vi "Script Find current Constants.vi"(8 "error in":errorcluster, 11 "Library in":refnum<vi>) -> (0 "error out":errorcluster, 1 "All Constant VIS":path[](array[path]), 2 "Constants Info":T1[](array[typedef]), 3 "Library out":refnum<vi>)   [LabVIEW 2020, in "ConstantErrorsMaker.lvlib"]
uses:
  ConstantErrorsMaker.lvlib
  Constant Info--cluster.ctl
  <vilib>/Utility/traverseref.llb/TRef TravTarget.ctl
  <vilib>/Utility/traverseref.llb/VI Scripting - Traverse.lvlib
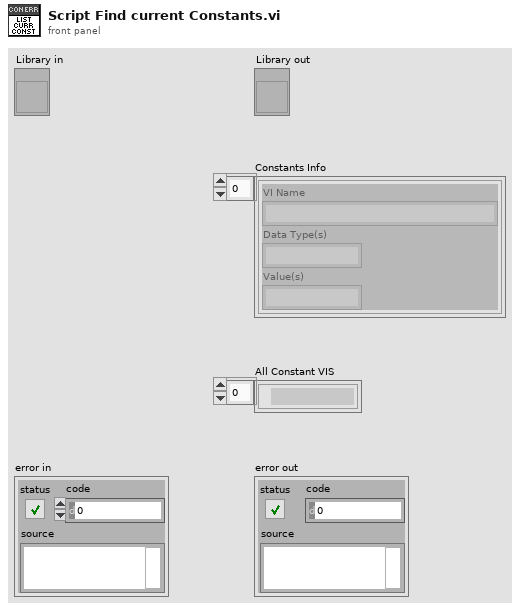
[diagram p1: front panel]
types:
  T1 = typedef "ConstantErrorsMaker.lvlib/Constant Info--cluster.ctl" = cluster{"VI Name":string, "Data Type(s)":string, "Value(s)":string}
  T2 = typedef "TRef TravTarget.ctl" = enum16{"FP", "BD", "Other"}
  T3 = typedef "NI_Data Type.lvlib/Data Type.ctl" = enum8{"Invalid Type", "Void", "I8", "I16", "I32", "I64", "U8", "U16", "U32", "U64", "Single Float", "Double Float", "Extended Float", "Single Complex", "Double Complex", "Extended Complex", "Enum U8", "Enum U16", "Enum U32", "Enum U64", "Single Float With Unit", "Double Float With Unit", "Extended Float With Unit", "Single Complex with Unit", "Double Complex with Unit", "Extended Complex with Unit", "Boolean", "String", "Path", "Picture", "Tag", "Array", "Cluster", "Variant", "LV Variant", "Waveform", "Timestamp", "Digital Waveform", "Digital Data", "ExpressData", "Refnum", "External Data", "VI", "Poly VI", "LabVIEW Class Instance", "Fixed Point", "Set Collection", "Map Collection"}
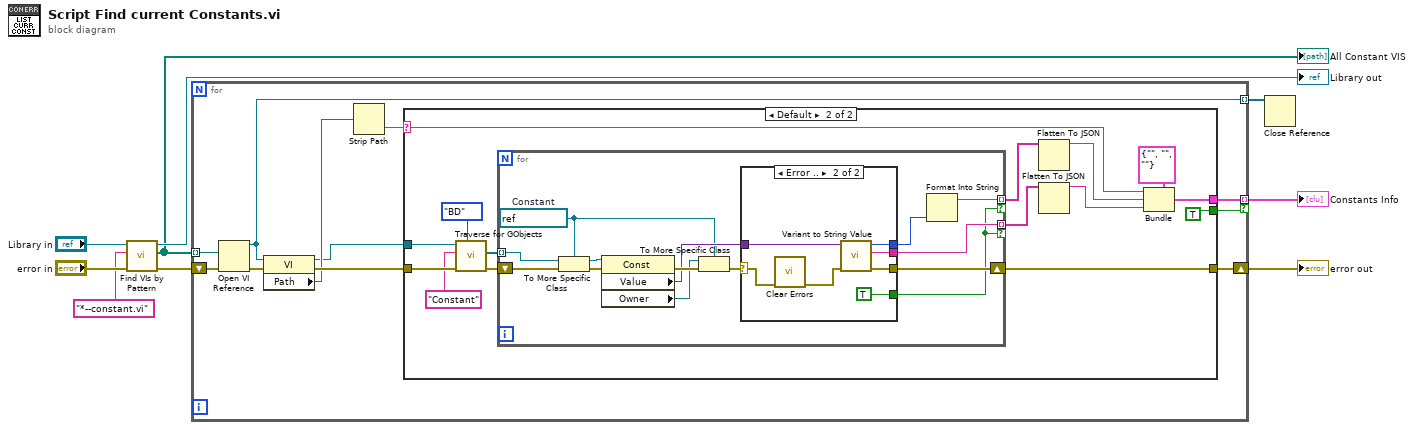
[diagram p0: block diagram]
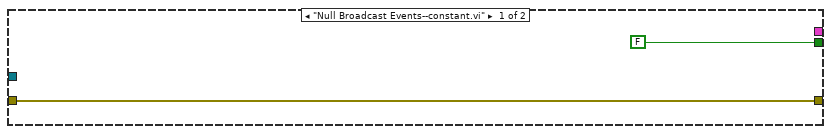
[diagram p2: hidden frame]
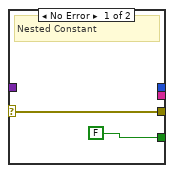
[diagram p3: hidden frame]
diagram:
  n1 = call "Find VIs by Pattern.vi"("error in"="error in", "pattern"="*--constant.vi", "Library in"="Library in") -> ("error out"=w7:errorcluster, "All Files in Dir"=w3:path[], "Library out"=→"Library out":refnum<vi>)  [unwired: 6 in]
  "All Constant VIS" <- w3
  n2 = for {
    tunnel: w3 -> [w16] mode=indexing
    shift-right: [w18] -> w8
    shift-left: w7 -> [w17]
    tunnel: [w12] -> w1 mode=indexing if=w10
    tunnel: [w11] -> w2 mode=indexing
    n3 = Open VI Reference(vi path=w16, error in (no error)=w17) -> (vi reference=w11:refnum<vi>, error out=w19:errorcluster)  [unwired: 4 in]
    n4 = property class="VI"(reference=w11, error in=w19) -> (reference out=w13:refnum<vi>, error out=w20:errorcluster, "Path"=w14:path)
    n5 = Strip Path(path=w14) -> (name=w15:string)  [unwired: 1 out]
    n6 = case shown="Default" w15 {
      selector: w15 -> [_ w34]
      tunnel: w20 -> [w22 w37]
      tunnel: [w22 w35] -> w18
      tunnel: w13 -> [_ w33]
      tunnel: [_ w29] -> w12
      tunnel: [FALSE TRUE] -> w10
      frame "Null Broadcast Events--constant.vi" {
      }
      frame Default {
        n7 = call <vilib>:"Traverse for GObjects.vi"("Traverse Target"=TRef_TravTarget."BD", "error in (no error)"=w37, "Class Name"="Constant", "VI Refnum"=w33) -> ("error out"=w36:errorcluster, "References"=w32:refnum<vi>[])  [unwired: 4 in, 2 out]
        n8 = for {
          shift-right: [w49] -> w35
          shift-left: w36 -> [w51]
          tunnel: w32 -> [w46] mode=indexing
          tunnel: [w43] -> w25 mode=indexing if=w40
          tunnel: [w39] -> w26 mode=indexing if=w40
          w41 = refnum<vi> refnum  # Constant
          n9 = To More Specific Class(target class=w41, reference=w46, error in=w51) -> (specific class reference=w45:refnum<vi>, error out=w50:errorcluster)
          n10 = property class="Const"(reference=w45, error in=w50) -> (error out=w48:errorcluster, "Value"=w44:variant, "Owner"=w42:refnum<vi>)  [unwired: 1 out]
          n11 = To More Specific Class(target class=w41, reference=w42, error in=w48) -> (error out=w47:errorcluster)  [unwired: 1 out]
          n12 = case shown="Error .." w47 {
            selector: w47 -> [w53 w60]
            tunnel: [w53 w58] -> w49
            tunnel: w44 -> [_ w56]
            tunnel: [_ w54] -> w43
            tunnel: [_ w55] -> w38
            tunnel: [FALSE TRUE] -> w40
            frame No Error {
              # "Nested Constant"
            }
            frame Error {
              n13 = call <vilib>:"Clear Errors.vi"("error in (no error)"=w60) -> ("error out"=w59:errorcluster)  [unwired: 5 in, 1 out]
              n14 = call "Variant to String Value.vi"("error in"=w59, "Value"=w56) -> ("error out"=w58:errorcluster, "String"=w54:string, "type"=w55:T3)  [unwired: 7 in]
            }
          }
          n15 = Format Into String(w38) -> (resulting string=w39:string)  [unwired: 3 in, 1 out]
        }
        n16 = Flatten To JSON(anything=w26) -> (JSON string=w24:string)  [unwired: 2 in, 1 out]
        n17 = Flatten To JSON(anything=w25) -> (JSON string=w23:string)  [unwired: 2 in, 1 out]
        n18 = Bundle(cluster=T1 {"VI Name"="", "Data Type(s)"="", "Value(s)"=""} ("output cluster"), "VI Name"=w34, "Data Type(s)"=w24, "Value(s)"=w23) -> (w29:T1)
      }
    }
  }
  "error out" <- w8
  "Constants Info" <- w1
  n19 = Close Reference(reference=w2) -> ()  [unwired: 1 in, 1 out]
